vi "BancadaCalib1.vi"() -> ()   [LabVIEW 2014]
uses:
  <vilib>/Analysis/baseanly.llb/Mean (DBL).vi
  <vilib>/Analysis/NI_AALBase.lvlib
panel:
  out "Waveform Graph":dynamicdata(graph)
  in  "Motor":bool
  out "Motor 2":bool
  out "Freio":bool
  in  "Freio 2":bool
  out "error out":errorcluster
  in  "factor 2":dbl
  out "km/h":dbl format="%#_4f"
  out "Freq":dbl
  out "RPM":dbl format="%#_4f"
  out "input lc (V)":dbl
  out "input tcB (V)":dbl
  out "input tcA (V)":dbl
  out "input ref (V)":dbl
  in  "factor":dbl
  out "hot B(mV)":dbl
  out "tc B(mV)":dbl
  out "tempB(degC)":dbl
  out "hot A(mV)":dbl
  out "tc A(mV)":dbl
  out "tempA(degC)":dbl
  out "temp Ref (degC)":dbl
  out "Force (Kgf)":dbl format="%#_4f"
  in  "offset":dbl step=0.01 format="%#_2f"
  in  "stop":bool
  out "Emf(Cold - mV)":dbl
  # "Cold Junction Information"
  # "Thermocouple A"
  # "Thermocouple B"
  # "Load Cell"
  # "RPM"
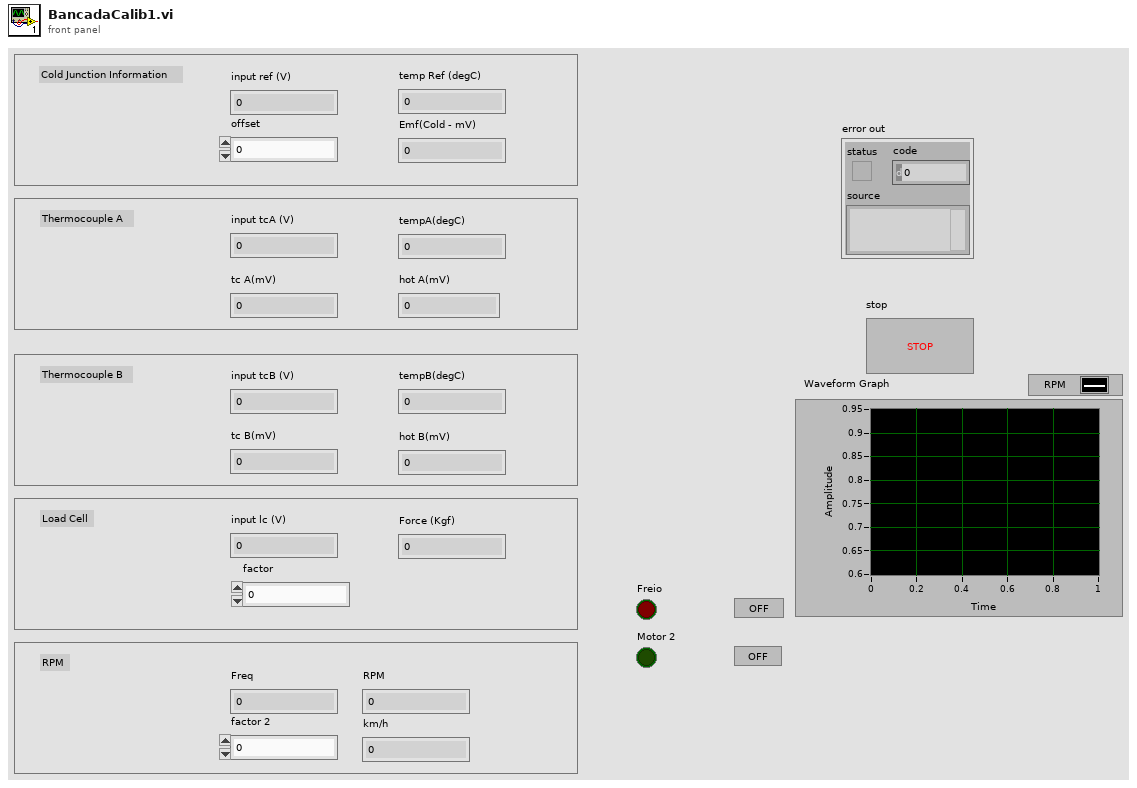
[diagram p1: front panel]
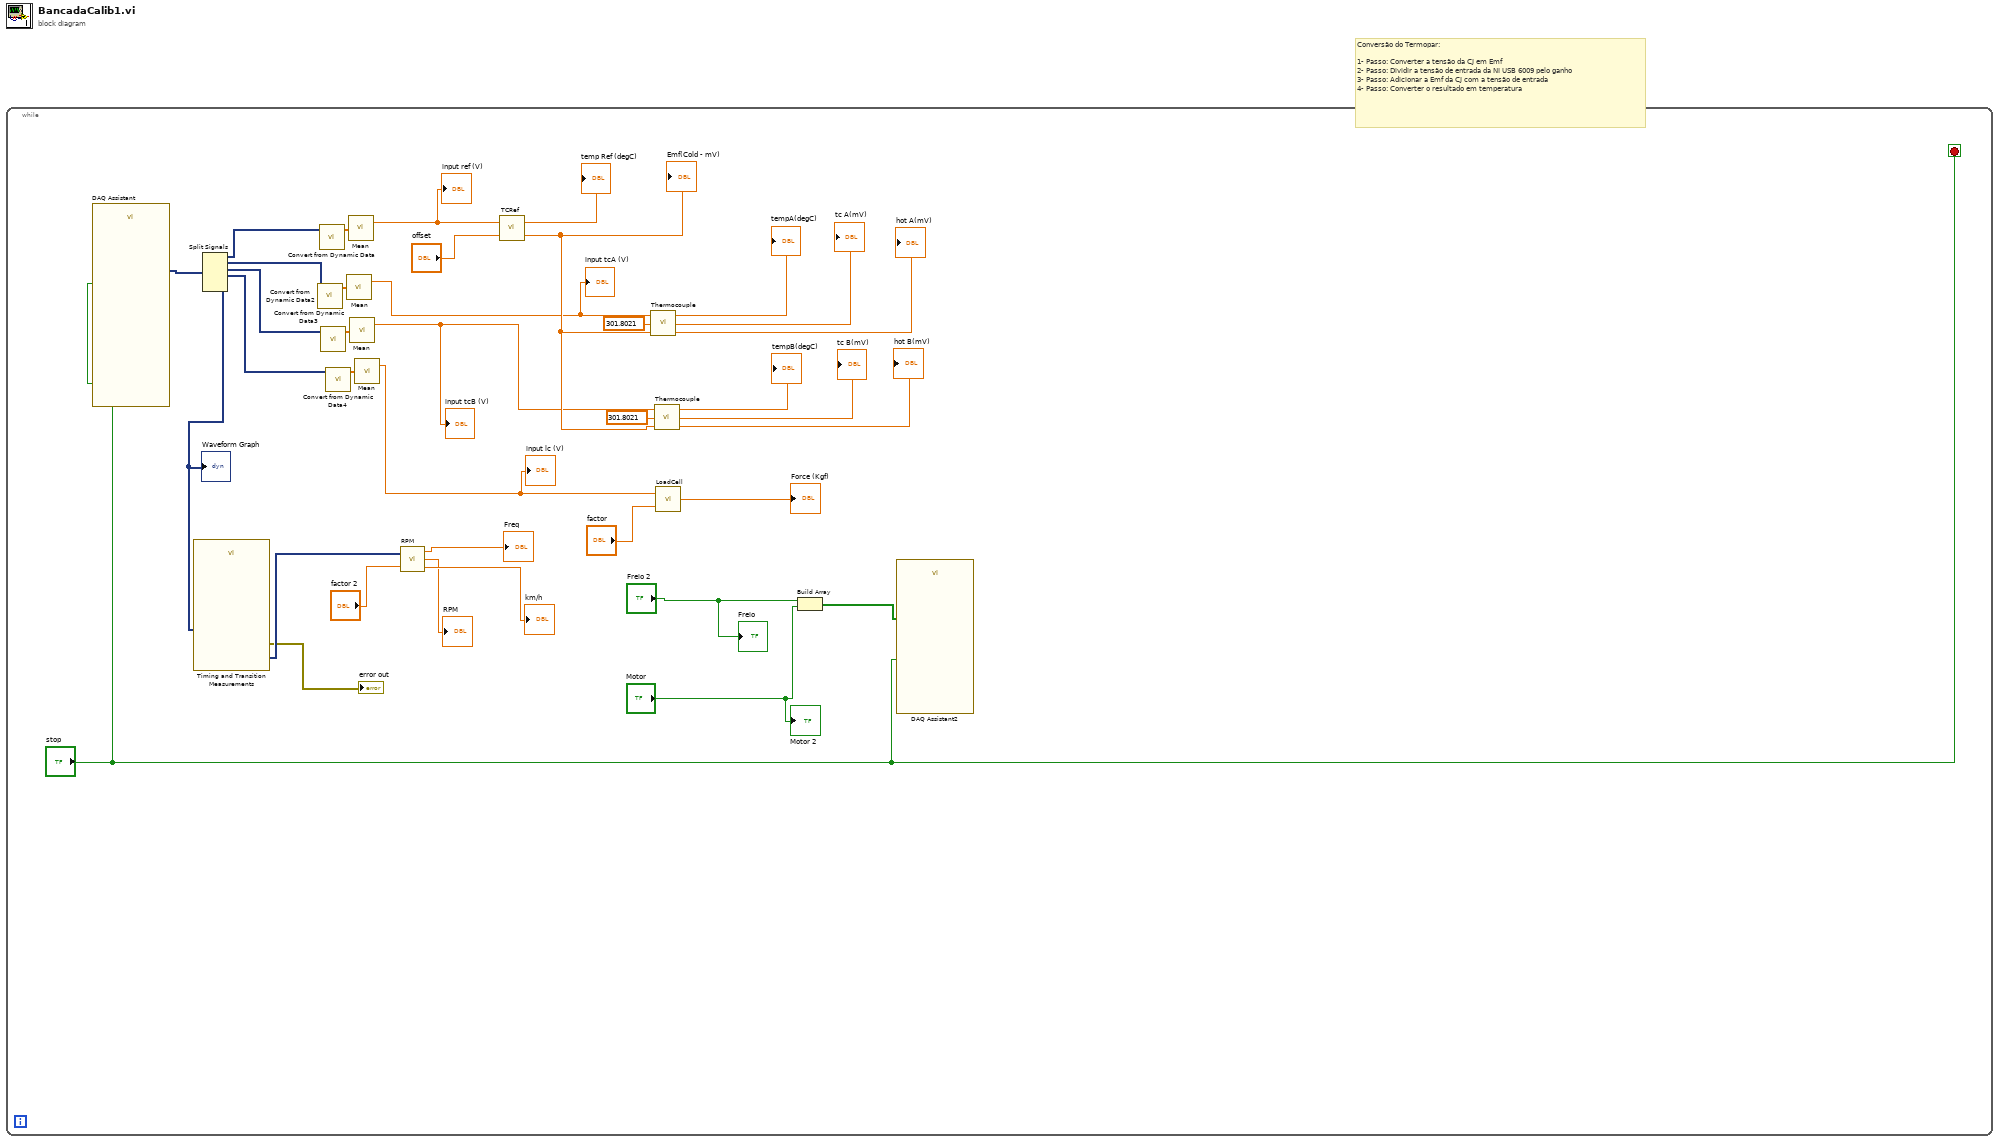
[diagram p0: block diagram]
diagram:
  # "Conversão do Termopar:\n\n1- Passo: Converter a tensão da CJ em Emf\n2- Passo: Dividir a tensão de entrada da NI USB 6009 pelo ganho\n3- Passo: Adicionar a Emf da CJ com a tensão de entrada\n4- Passo: Converter o resultado em temperatura"
  n1 = while {
    stop <- "stop" stop-if-true
    n2 = call "DAQ Assistant"("stop (F)"="stop") -> ("data"=w16:dynamicdata)  [unwired: 15 in, 3 out]
    n3 = Split Signals(w16) -> (w13:dynamicdata, w11:dynamicdata, w9:dynamicdata, w7:dynamicdata, w5:dynamicdata)  [unwired: 6 in, 1 out]
    "Waveform Graph" <- w5
    n4 = call "Timing and Transition Measurements"("Signals"=w5) -> ("error out"=→"error out":errorcluster, "Frequency"=w15:dynamicdata)  [unwired: 9 in]
    n5 = call "Convert from Dynamic Data2"("Dynamic Data Type"=w11) -> ("Array"=w10:dbl[])  [unwired: 3 in]
    n6 = call "Convert from Dynamic Data"("Dynamic Data Type"=w13) -> ("Array"=w12:dbl[])  [unwired: 3 in]
    n7 = call "Convert from Dynamic Data3"("Dynamic Data Type"=w9) -> ("Array"=w8:dbl[])  [unwired: 3 in]
    n8 = call "Convert from Dynamic Data4"("Dynamic Data Type"=w7) -> ("Array"=w6:dbl[])  [unwired: 3 in]
    n9 = call-poly <vilib>:"Mean.vi"("X"=w10) -> ("mean"=w23:dbl)  [unwired: 1 out]
    "input tcA (V)" <- w23
    n10 = call-poly <vilib>:"Mean.vi"("X"=w12) -> ("mean"=w24:dbl)  [unwired: 1 out]
    "input ref (V)" <- w24
    n11 = call-poly <vilib>:"Mean.vi"("X"=w8) -> ("mean"=w21:dbl)  [unwired: 1 out]
    "input tcB (V)" <- w21
    n12 = call-poly <vilib>:"Mean.vi"("X"=w6) -> ("mean"=w22:dbl)  [unwired: 1 out]
    "input lc (V)" <- w22
    n13 = call "RPM.vi"("data"=w15, "factor"="factor 2") -> ("Frequency"=→"Freq":dbl, "RPM"=→"RPM":dbl, "km/h"=→"km/h":dbl)
    n14 = call "TCRef.vi"("offset"="offset", "data"=w24) -> ("emf(mV)"=w30:dbl, "temp (degC)"=→"temp Ref (degC)":dbl)
    "Emf(Cold - mV)" <- w30
    n15 = call "Thermocouple.vi"("cj(mV)"=w30, "factor"=301.8021, "data"=w23) -> ("hot(mV)"=→"hot A(mV)":dbl, "tc(mV)"=→"tc A(mV)":dbl, "temp(degC)"=→"tempA(degC)":dbl)
    n16 = call "Thermocouple.vi"("cj(mV)"=w30, "factor"=301.8021, "data"=w21) -> ("hot(mV)"=→"hot B(mV)":dbl, "tc(mV)"=→"tc B(mV)":dbl, "temp(degC)"=→"tempB(degC)":dbl)
    n17 = call "LoadCell.vi"("factor"="factor", "data"=w22) -> ("force (Kgf)"=→"Force (Kgf)":dbl)
    n18 = Build Array("Freio 2", "Motor") -> (w3:bool[])
    n19 = call "DAQ Assistant2"("data"=w3, "stop (T)"="stop") -> ()  [unwired: 16 in, 2 out]
    "Freio" <- "Freio 2"
    "Motor 2" <- "Motor"
  }
